vi "inclineCheck.vi"() -> ()   [LabVIEW 2018]
panel:
  out "Array":dbl[](array[numeric])
  out "String to Array":string[](array[string])
  out "Press":bool
  out "Quickincline":bool
  out "Incline":dbl(graph)
  out "Press Next":dbl
  out "MAX":dbl
  out "MIN":dbl
  out "negative incline":dbl
  in  "EQF1259 com port":refnum<visa-resource-name>
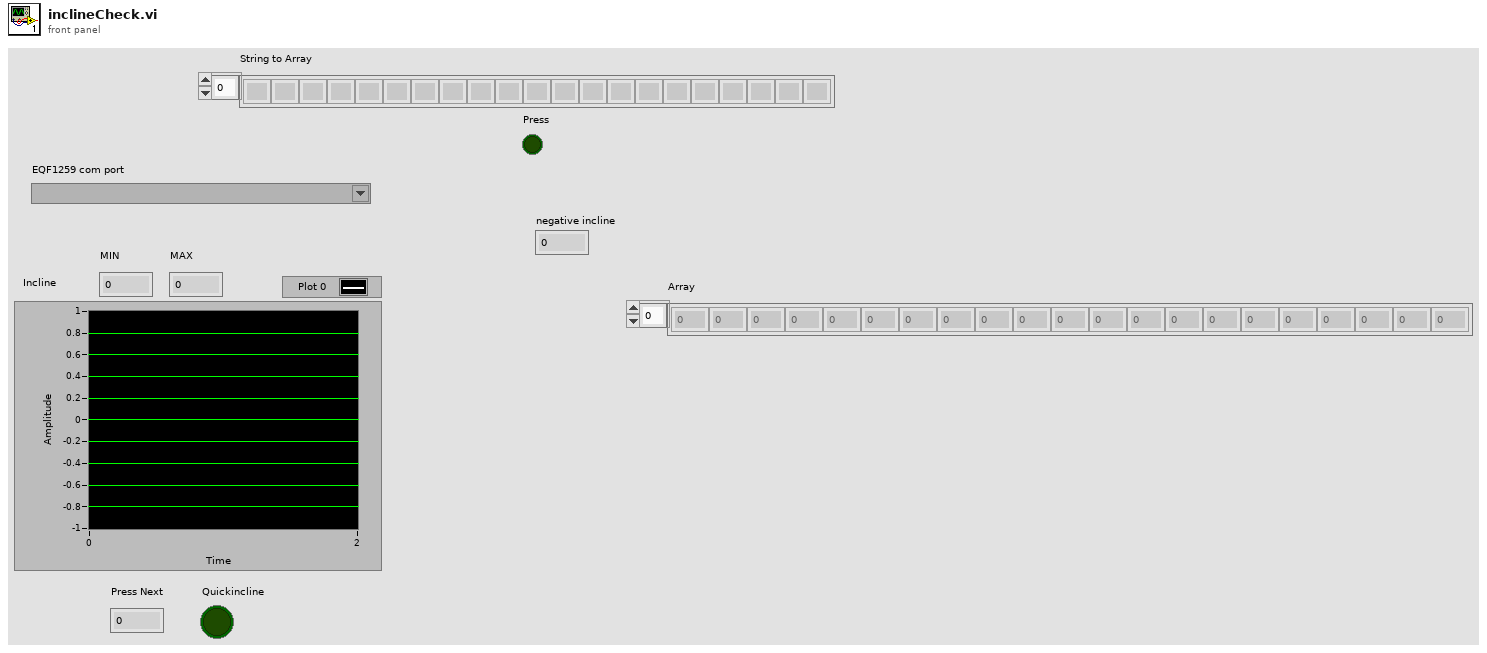
[diagram p1: front panel]
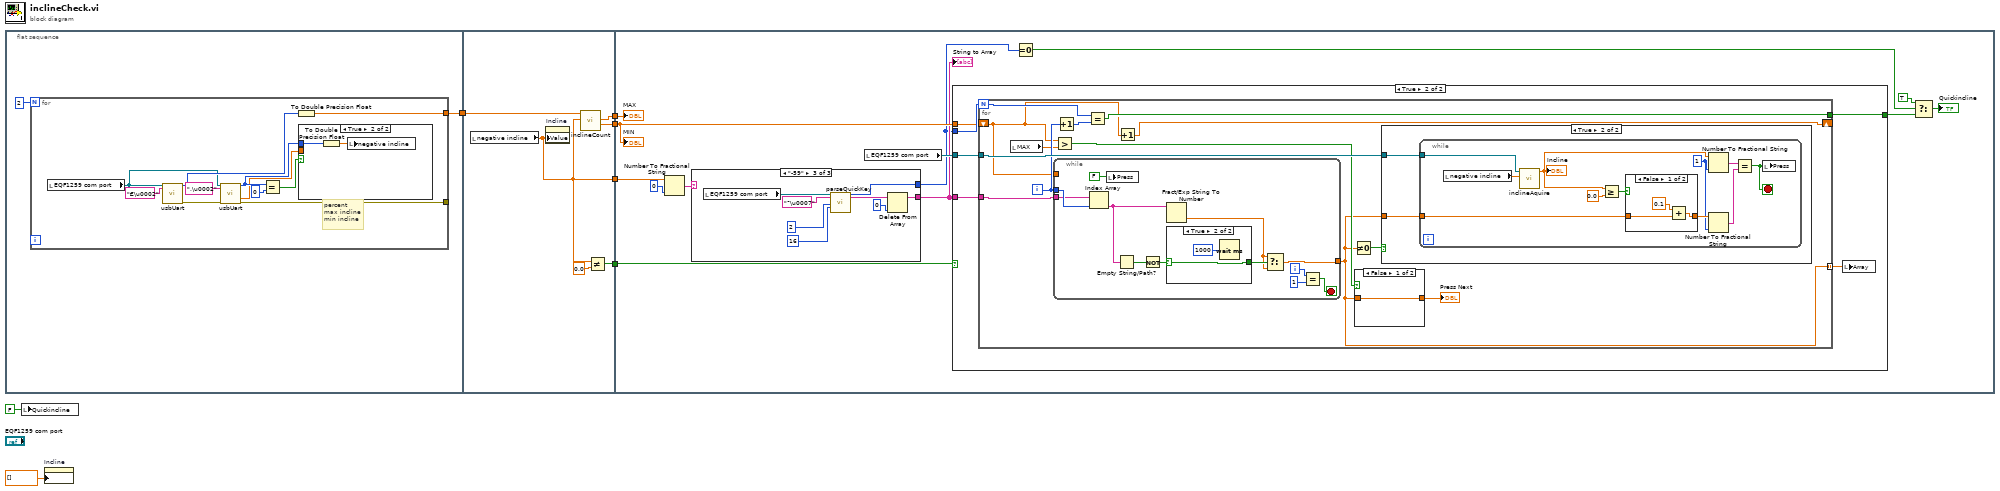
[diagram p0: block diagram]
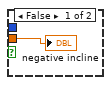
[diagram p2: hidden frame]
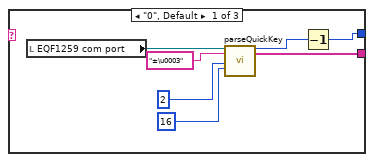
[diagram p3: hidden frame]
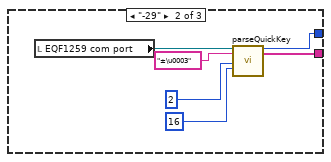
[diagram p4: hidden frame]
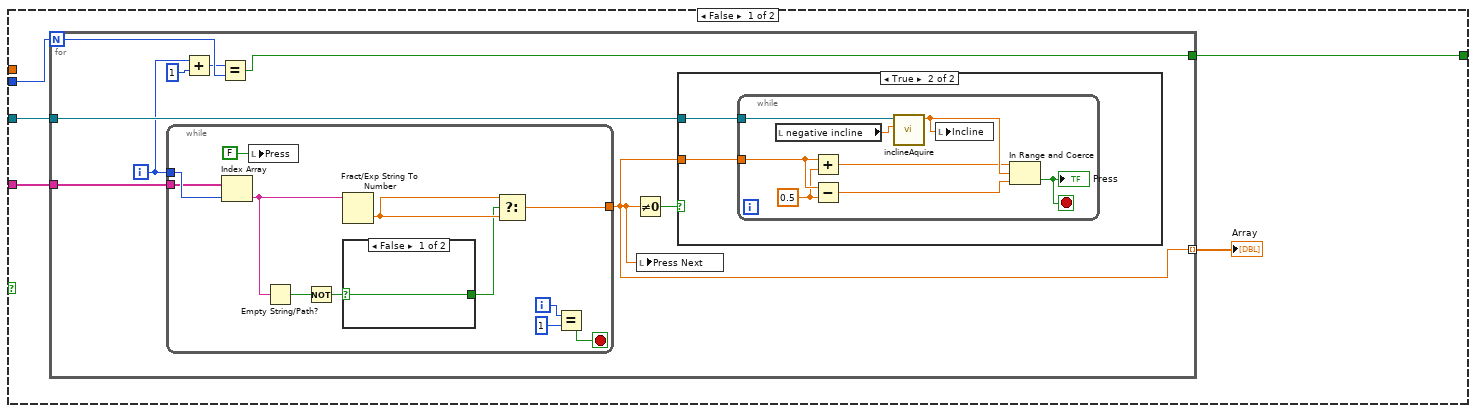
[diagram p5: hidden frame]
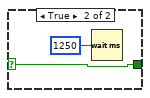
[diagram p7: hidden frame]
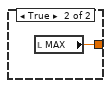
[diagram p10: hidden frame]
diagram:
  n1 = flat-sequence {
    tunnel: [w8] -> w7
    tunnel: [w27] -> w6
    tunnel: [w28] -> w5
    tunnel: [w25] -> w4
    tunnel: w7 -> [w26]
    tunnel: [w24] -> w2
    tunnel: w6 -> [w35]
    tunnel: w5 -> [w42]
    tunnel: w4 -> [w40]
    tunnel: w2 -> [w32]
    frame #0 {
      n2 = for {
        N: 2 -> [_]
        tunnel: [w11] -> _
        tunnel: [w10] -> w8
        # "percent\nmax incline\nmin incline"
        n3 = local read "EQF1259 com port"() -> (w13:refnum<visa-resource-name>)
        n4 = call "usbUart.vi"("VISA resource name"=w13, "write buffer"="€\u0002") -> ("number[0]"=w19:u32, "error out"=w12:errorcluster)  [unwired: 2 in, 14 out]
        n5 = call "usbUart.vi"("VISA resource name"=w13, "write buffer"="‚\u0002", "error in (no error)"=w12) -> ("number[0]"=w15:u32, "negative incline"=w14:dbl, "error out"=w11:errorcluster)  [unwired: 1 in, 13 out]
        n6 = Equal?(x=w15, y=u32 0) -> (x = y?=w16:bool)
        n7 = To Double Precision Float(number=w19) -> (double precision float=w10:dbl)
        n8 = case shown="True" w16 {
          tunnel: w15 -> [_ w23]
          tunnel: w14 -> [w21 _]
          frame False {
            "negative incline" <- w21
          }
          frame True {
            n9 = To Double Precision Float(number=w23) -> (double precision float=w22:dbl)
            n10 = local write "negative incline"(w22) -> ()
          }
        }
      }
    }
    frame #1 {
      n11 = local read "negative incline"() -> (w24:dbl)
      n12 = property on="Incline" class="WFChart (strict)"("Value"=w24) -> ()  [unwired: 2 in, 2 out]
      n13 = call "inclineCount.vi"("negative incline"=w24, "max incline"=w26) -> ("press start"=w27:dbl, "max incline"=w25:dbl)  [unwired: 6 in, 2 out]
      n14 = Not Equal?(x=w24, y=0.0) -> (x != y?=w28:bool)
    }
    frame #2 {
      n15 = Number To Fractional String(number=w32, precision (6)=i16 0) -> (F-format string=w31:string)  [unwired: 2 in]
      n16 = case shown="\"-59\"" w31 {
        tunnel: [w43 w52 w56] -> w34
        tunnel: [w47 w55 w60] -> w33
        frame "0", Default {
          n17 = local read "EQF1259 com port"() -> (w49:refnum<visa-resource-name>)
          n18 = call "parseQuickKey.vi"("VISA resource name"=w49, "write buffer"="±\u0003", "y"=2, "x"=16) -> ("lengthString"=w44:i32, "KeyCodeName"=w43:string[])  [unwired: 11 in, 3 out]
          n19 = Decrement(x=w44) -> (x-1=w47:i32)
        }
        frame "-29" {
          n20 = local read "EQF1259 com port"() -> (w53:refnum<visa-resource-name>)
          n21 = call "parseQuickKey.vi"("VISA resource name"=w53, "write buffer"="±\u0003", "y"=2, "x"=16) -> ("lengthString"=w55:i32, "KeyCodeName"=w52:string[])  [unwired: 11 in, 3 out]
        }
        frame "-59" {
          n22 = local read "EQF1259 com port"() -> (w63:refnum<visa-resource-name>)
          n23 = call "parseQuickKey.vi"("VISA resource name"=w63, "write buffer"="¯\u0007", "y"=2, "x"=16) -> ("lengthString"=w60:i32, "KeyCodeName"=w57:string[])  [unwired: 11 in, 3 out]
          n24 = Delete From Array(array=w57, index=0) -> (array with subset deleted=w56:string[])  [unwired: 1 in, 1 out]
        }
      }
      "String to Array" <- w34
      n25 = local read "EQF1259 com port"() -> (w41:refnum<visa-resource-name>)
      n26 = case shown="True" w42 {
        tunnel: [w67 w108] -> w39
        tunnel: w33 -> [w68 w107]
        tunnel: w41 -> [w66 w106]
        tunnel: w35 -> [_ w105]
        tunnel: w34 -> [w65 w104]
        frame False {
          n27 = for {
            N: w68 -> [w76]
            tunnel: [w75] -> w67
            tunnel: w66 -> [w73]
            tunnel: w65 -> [w71]
            tunnel: [w70] -> w64 mode=indexing
            i -> [w72]
            n28 = while {
              tunnel: [w99] -> w70
              tunnel: w72 -> [w98]
              tunnel: w71 -> [w94]
              i -> [w95]
              stop <- w96 stop-if-true
              n29 = Index Array(array=w94, index=w98) -> (element=w93:string)
              n30 = local write "Press"(FALSE ("Press")) -> ()
              n31 = Empty String/Path?(string/path=w93) -> (empty?=w91:bool)
              n32 = Not(x=w91) -> (.not. x?=w89:bool)
              n33 = Fract/Exp String To Number(string=w93) -> (number=w92:dbl)  [unwired: 3 in, 1 out]
              n34 = case shown="False" w89 {
                selector: w89 -> [w100 w101]
                tunnel: [w100 w101] -> w88
                frame False {
                }
                frame True {
                  n35 = Wait (ms)(milliseconds to wait=u32 1250) -> ()  [unwired: 1 out]
                }
              }
              n36 = Select(t=w92, s=w88, f=w92) -> (s? t:f=w99:dbl)
              n37 = Equal?(x=w95, y=1) -> (x = y?=w96:bool)
            }
            n38 = Add(x=w72, y=1) -> (x+y=w74:i32)
            n39 = Equal?(x=w74, y=w76) -> (x = y?=w75:bool)
            n40 = Not Equal To 0?(x=w70) -> (x != 0?=w69:bool)
            n41 = local write "Press Next"(w70) -> ()
            n42 = case shown="True" w69 {
              tunnel: w73 -> [_ w79]
              tunnel: w70 -> [_ w78]
              frame False {
              }
              frame True {
                n43 = while {
                  tunnel: w79 -> [w86]
                  tunnel: w78 -> [w82]
                  stop <- w83 stop-if-true
                  w80 = 0.5 ("y")
                  n44 = local read "negative incline"() -> (w87:dbl)
                  n45 = Add(x=w82, y=w80) -> (x+y=w81:dbl)
                  n46 = Subtract(x=w82, y=w80) -> (x-y=w84:dbl)
                  n47 = call "inclineAquire.vi"("Negative Incline"=w87, "VISA Refnum in"=w86) -> ("Incline Out"=w85:dbl)  [unwired: 8 in, 1 out]
                  n48 = local write "Incline"(w85) -> ()
                  n49 = In Range and Coerce(upper limit=w81, x=w85, lower limit=w84) -> (In Range?=w83:bool)  [unwired: 1 out]
                  "Press" <- w83
                }
              }
            }
          }
          "Array" <- w64
        }
        frame True {
          n50 = for {
            N: w107 -> [w119]
            tunnel: w106 -> [w121]
            tunnel: [w120] -> w108
            shift-right: [w116] -> _
            shift-left: w105 -> [w114]
            tunnel: w104 -> [w117]
            tunnel: [w110] -> w103 mode=indexing
            i -> [w118]
            n51 = local read "MAX"() -> (w113:dbl)
            n52 = while {
              tunnel: [w152] -> w110
              tunnel: w118 -> [w151]
              tunnel: w114 -> [_]
              tunnel: w117 -> [w147]
              i -> [w148]
              stop <- w149 stop-if-true
              n53 = Index Array(array=w147, index=w151) -> (element=w144:string)
              n54 = local write "Press"(FALSE ("Press")) -> ()
              n55 = Empty String/Path?(string/path=w144) -> (empty?=w142:bool)
              n56 = Not(x=w142) -> (.not. x?=w145:bool)
              n57 = Fract/Exp String To Number(string=w144) -> (number=w143:dbl)  [unwired: 3 in, 1 out]
              n58 = case shown="True" w145 {
                selector: w145 -> [w153 w154]
                tunnel: [w153 w154] -> w146
                frame False {
                }
                frame True {
                  n59 = Wait (ms)(milliseconds to wait=u32 1000) -> ()  [unwired: 1 out]
                }
              }
              n60 = Select(t=w143, s=w146, f=w143) -> (s? t:f=w152:dbl)
              n61 = Equal?(x=w148, y=1) -> (x = y?=w149:bool)
            }
            n62 = Greater?(x=w114, y=w113) -> (0:w115:bool)
            n63 = Increment(x=w118) -> (x+1=w111:i32)
            n64 = Equal?(x=w119, y=w111) -> (x = y?=w120:bool)
            n65 = Increment(x=w114) -> (x+1=w116:dbl)
            n66 = Not Equal To 0?(x=w110) -> (x != 0?=w109:bool)
            n67 = case shown="False" w115 {
              tunnel: [w139 w140] -> w112
              tunnel: w110 -> [w139 _]
              frame False {
              }
              frame True {
                n68 = local read "MAX"() -> (w140:dbl)
              }
            }
            "Press Next" <- w112
            n69 = case shown="True" w109 {
              tunnel: w121 -> [_ w123]
              tunnel: w110 -> [_ w122]
              frame False {
              }
              frame True {
                n70 = while {
                  tunnel: w123 -> [w134]
                  tunnel: w122 -> [w124]
                  stop <- w125 stop-if-true
                  w128 = i16 1 ("precision (6)")
                  n71 = local read "negative incline"() -> (w133:dbl)
                  n72 = call "inclineAquire.vi"("Negative Incline"=w133, "VISA Refnum in"=w134) -> ("Incline Out"=w130:dbl)  [unwired: 8 in, 1 out]
                  "Incline" <- w130
                  n73 = Greater Or Equal?(x=w130, y=0.0) -> (x >= y?=w132:bool)
                  n74 = case shown="False" w132 {
                    tunnel: w124 -> [w136 w138]
                    tunnel: [w135 w138] -> w129
                    frame False {
                      n75 = Add(x=0.1, y=w136) -> (x+y=w135:dbl)
                    }
                    frame True {
                    }
                  }
                  n76 = Number To Fractional String(number=w130, precision (6)=w128) -> (F-format string=w126:string)  [unwired: 2 in]
                  n77 = Number To Fractional String(number=w129, precision (6)=w128) -> (F-format string=w127:string)  [unwired: 2 in]
                  n78 = Equal?(x=w126, y=w127) -> (x = y?=w125:bool)
                  n79 = local write "Press"(w125) -> ()
                }
              }
            }
          }
          n80 = local write "Array"(w103) -> ()
        }
      }
      n81 = Equal To 0?(x=w33) -> (x = 0?=w37:bool)
      n82 = Select(t=TRUE, s=w37, f=w39) -> (s? t:f=→"Quickincline":bool)
      "MAX" <- w40
      "MIN" <- w35
    }
  }
  n83 = local write "Quickincline"(FALSE ("Quickincline")) -> ()
  n84 = property on="Incline" class="WFChart (strict)"("History Data"=dbl[] []) -> ()  [unwired: 2 in, 2 out]
